vi "校准参数读取.vi"(8 "error in":errorcluster caption="错误输入", 11 "Channel":u16=81 format="%.0x") -> (0 "error out":errorcluster caption="错误输出", 1 "斜率":i32, 2 "截距":i32)   [LabVIEW 2020]
uses:
  D/Program Files (x86)/National Instruments/LabVIEW 2020/user.lib/PCANBasic/PCANBasic.lvlib
panel:
  out "function return 4":u32 format="%.0x"
  out "function return 3":u32 format="%.0x"
  out "function return 2":u32 format="%.0x"
  out "function return":u32 format="%.0x"
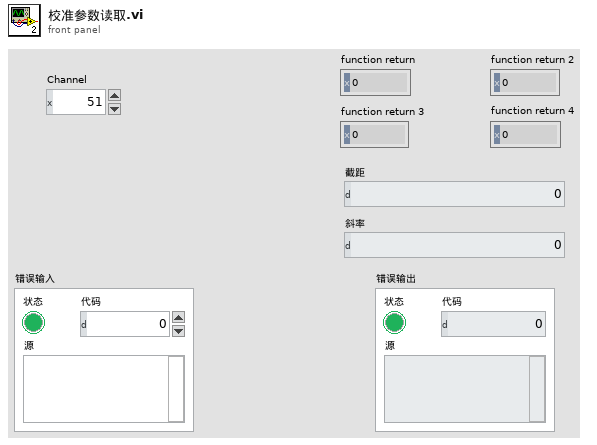
[diagram p1: front panel]
types:
  T1 = cluster{"ID":u32, "MSGTYPE":u8, "DLC":u8, "DATA[0]":u8, "DATA[1]":u8, "DATA[2]":u8, "DATA[3]":u8, "DATA[4]":u8, "DATA[5]":u8, "DATA[6]":u8, "DATA[7]":u8, "DATA[8]":u8, "DATA[9]":u8, "DATA[10]":u8, "DATA[11]":u8, "DATA[12]":u8, "DATA[13]":u8, "DATA[14]":u8, "DATA[15]":u8, "DATA[16]":u8, "DATA[17]":u8, "DATA[18]":u8, "DATA[19]":u8, "DATA[20]":u8, "DATA[21]":u8, "DATA[22]":u8, "DATA[23]":u8, "DATA[24]":u8, "DATA[25]":u8, "DATA[26]":u8, "DATA[27]":u8, "DATA[28]":u8, "DATA[29]":u8, "DATA[30]":u8, "DATA[31]":u8, "DATA[32]":u8, "DATA[33]":u8, "DATA[34]":u8, "DATA[35]":u8, "DATA[36]":u8, "DATA[37]":u8, "DATA[38]":u8, "DATA[39]":u8, "DATA[40]":u8, "DATA[41]":u8, "DATA[42]":u8, "DATA[43]":u8, "DATA[44]":u8, "DATA[45]":u8, "DATA[46]":u8, "DATA[47]":u8, "DATA[48]":u8, "DATA[49]":u8, "DATA[50]":u8, "DATA[51]":u8, "DATA[52]":u8, "DATA[53]":u8, "DATA[54]":u8, "DATA[55]":u8, "DATA[56]":u8, "DATA[57]":u8, "DATA[58]":u8, "DATA[59]":u8, "DATA[60]":u8, "DATA[61]":u8, "DATA[62]":u8, "DATA[63]":u8}
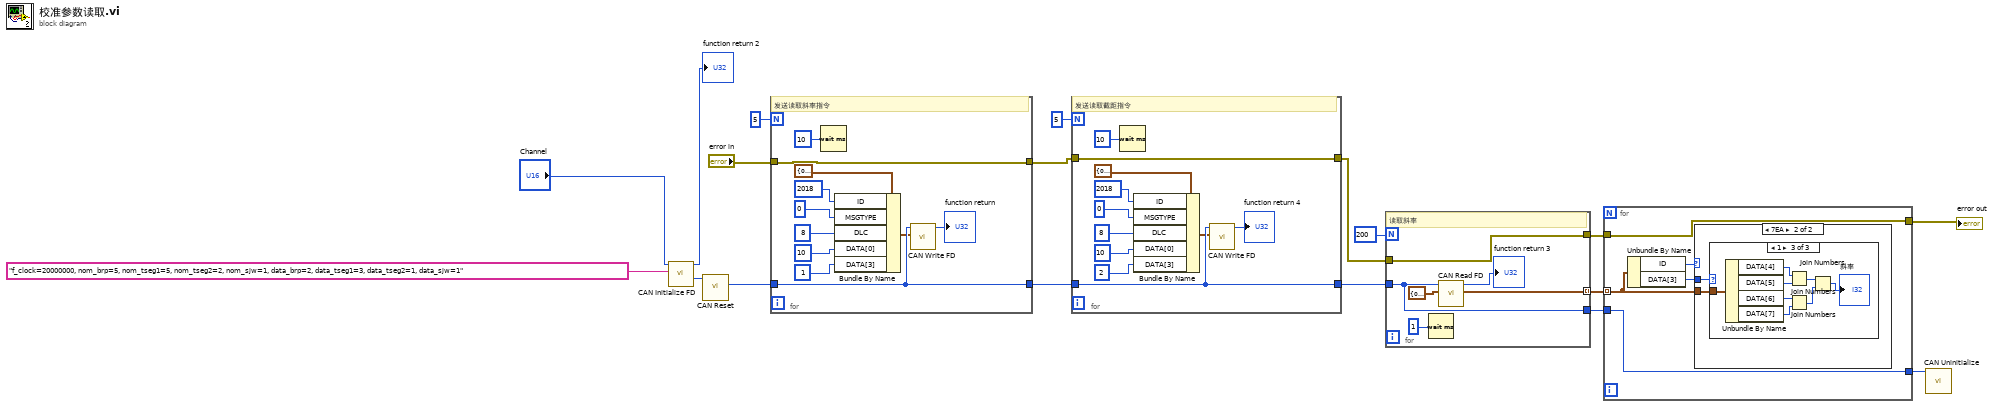
[diagram p0: block diagram]
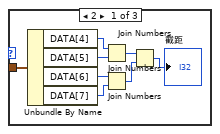
[diagram p3: hidden frame]
diagram:
  n1 = call "CAN Initialize FD.vi"("BitrateFD"="f_clock=20000000, nom_brp=5, nom_tseg1=5, nom_tseg2=2, nom_sjw=1, data_brp=2, data_tseg1=3, data_tseg2=1, data_sjw=1", "Channel"="Channel") -> ("Channel out"=w10:u16, "function return"=→"function return 2":u32)  [unwired: 7 in, 1 out]
  n2 = call "CAN Reset.vi"("Channel in"=w10) -> ("Channel out"=w9:u16)  [unwired: 9 in, 1 out]
  n3 = for {
    N: 5 -> [_]
    tunnel: w9 -> [w26]
    tunnel: [w26] -> w8
    tunnel: "error in" -> [w19]
    tunnel: [w19] -> w4
    # "发送读取斜率指令"
    n4 = Wait (ms)(milliseconds to wait=u32 10 ("等待时间（毫秒）")) -> ()  [unwired: 1 out]
    n5 = Bundle By Name(cluster=T1 {"ID"=0, "MSGTYPE"=0, "DLC"=0, "DATA[0]"=0, "DATA[1]"=0, "DATA[2]"=0, "DATA[3]"=0, "DATA[4]"=0, "DATA[5]"=0, "DATA[6]"=0, "DATA[7]"=0, "DATA[8]"=0, "DATA[9]"=0, "DATA[10]"=0, "DATA[11]"=0, "DATA[12]"=0, "DATA[13]"=0, "DATA[14]"=0, "DATA[15]"=0, "DATA[16]"=0, "DATA[17]"=0, "DATA[18]"=0, "DATA[19]"=0, "DATA[20]"=0, "DATA[21]"=0, "DATA[22]"=0, "DATA[23]"=0, "DATA[24]"=0, "DATA[25]"=0, "DATA[26]"=0, "DATA[27]"=0, "DATA[28]"=0, "DATA[29]"=0, "DATA[30]"=0, "DATA[31]"=0, "DATA[32]"=0, "DATA[33]"=0, "DATA[34]"=0, "DATA[35]"=0, "DATA[36]"=0, "DATA[37]"=0, "DATA[38]"=0, "DATA[39]"=0, "DATA[40]"=0, "DATA[41]"=0, "DATA[42]"=0, "DATA[43]"=0, "DATA[44]"=0, "DATA[45]"=0, "DATA[46]"=0, "DATA[47]"=0, "DATA[48]"=0, "DATA[49]"=0, "DATA[50]"=0, "DATA[51]"=0, "DATA[52]"=0, "DATA[53]"=0, "DATA[54]"=0, "DATA[55]"=0, "DATA[56]"=0, "DATA[57]"=0, "DATA[58]"=0, "DATA[59]"=0, "DATA[60]"=0, "DATA[61]"=0, "DATA[62]"=0, "DATA[63]"=0} ("MessageBuffer"), "ID"=u32 2018, "MSGTYPE"=u8 0, "DLC"=u8 8 ("ID"), "DATA[0]"=u8 10 ("ID"), "DATA[3]"=u8 1) -> (w20:T1)
    n6 = call "CAN Write FD.vi"("MessageBuffer"=w20, "Channel"=w26) -> ("function return"=→"function return":u32)  [unwired: 7 in, 2 out]
  }
  n7 = for {
    N: 5 -> [_]
    tunnel: w8 -> [w37]
    tunnel: [w37] -> w7
    tunnel: w4 -> [w30]
    tunnel: [w30] -> w3
    # "发送读取截距指令"
    n8 = Wait (ms)(milliseconds to wait=u32 10 ("等待时间（毫秒）")) -> ()  [unwired: 1 out]
    n9 = Bundle By Name(cluster=T1 {"ID"=0, "MSGTYPE"=0, "DLC"=0, "DATA[0]"=0, "DATA[1]"=0, "DATA[2]"=0, "DATA[3]"=0, "DATA[4]"=0, "DATA[5]"=0, "DATA[6]"=0, "DATA[7]"=0, "DATA[8]"=0, "DATA[9]"=0, "DATA[10]"=0, "DATA[11]"=0, "DATA[12]"=0, "DATA[13]"=0, "DATA[14]"=0, "DATA[15]"=0, "DATA[16]"=0, "DATA[17]"=0, "DATA[18]"=0, "DATA[19]"=0, "DATA[20]"=0, "DATA[21]"=0, "DATA[22]"=0, "DATA[23]"=0, "DATA[24]"=0, "DATA[25]"=0, "DATA[26]"=0, "DATA[27]"=0, "DATA[28]"=0, "DATA[29]"=0, "DATA[30]"=0, "DATA[31]"=0, "DATA[32]"=0, "DATA[33]"=0, "DATA[34]"=0, "DATA[35]"=0, "DATA[36]"=0, "DATA[37]"=0, "DATA[38]"=0, "DATA[39]"=0, "DATA[40]"=0, "DATA[41]"=0, "DATA[42]"=0, "DATA[43]"=0, "DATA[44]"=0, "DATA[45]"=0, "DATA[46]"=0, "DATA[47]"=0, "DATA[48]"=0, "DATA[49]"=0, "DATA[50]"=0, "DATA[51]"=0, "DATA[52]"=0, "DATA[53]"=0, "DATA[54]"=0, "DATA[55]"=0, "DATA[56]"=0, "DATA[57]"=0, "DATA[58]"=0, "DATA[59]"=0, "DATA[60]"=0, "DATA[61]"=0, "DATA[62]"=0, "DATA[63]"=0} ("MessageBuffer"), "ID"=u32 2018, "MSGTYPE"=u8 0, "DLC"=u8 8 ("ID"), "DATA[0]"=u8 10 ("ID"), "DATA[3]"=u8 2) -> (w31:T1)
    n10 = call "CAN Write FD.vi"("MessageBuffer"=w31, "Channel"=w37) -> ("function return"=→"function return 4":u32)  [unwired: 7 in, 2 out]
  }
  n11 = for {
    N: 200 -> [_]
    tunnel: w7 -> [w45]
    tunnel: [w44] -> w16 mode=indexing
    tunnel: [w45] -> w15
    tunnel: w3 -> [w41]
    tunnel: [w41] -> w2
    # "读取斜率"
    n12 = Wait (ms)(milliseconds to wait=u32 1 ("等待时间（毫秒）")) -> ()  [unwired: 1 out]
    n13 = call "CAN Read FD.vi"("MessageBuffer"=T1 {"ID"=0, "MSGTYPE"=0, "DLC"=0, "DATA[0]"=0, "DATA[1]"=0, "DATA[2]"=0, "DATA[3]"=0, "DATA[4]"=0, "DATA[5]"=0, "DATA[6]"=0, "DATA[7]"=0, "DATA[8]"=0, "DATA[9]"=0, "DATA[10]"=0, "DATA[11]"=0, "DATA[12]"=0, "DATA[13]"=0, "DATA[14]"=0, "DATA[15]"=0, "DATA[16]"=0, "DATA[17]"=0, "DATA[18]"=0, "DATA[19]"=0, "DATA[20]"=0, "DATA[21]"=0, "DATA[22]"=0, "DATA[23]"=0, "DATA[24]"=0, "DATA[25]"=0, "DATA[26]"=0, "DATA[27]"=0, "DATA[28]"=0, "DATA[29]"=0, "DATA[30]"=0, "DATA[31]"=0, "DATA[32]"=0, "DATA[33]"=0, "DATA[34]"=0, "DATA[35]"=0, "DATA[36]"=0, "DATA[37]"=0, "DATA[38]"=0, "DATA[39]"=0, "DATA[40]"=0, "DATA[41]"=0, "DATA[42]"=0, "DATA[43]"=0, "DATA[44]"=0, "DATA[45]"=0, "DATA[46]"=0, "DATA[47]"=0, "DATA[48]"=0, "DATA[49]"=0, "DATA[50]"=0, "DATA[51]"=0, "DATA[52]"=0, "DATA[53]"=0, "DATA[54]"=0, "DATA[55]"=0, "DATA[56]"=0, "DATA[57]"=0, "DATA[58]"=0, "DATA[59]"=0, "DATA[60]"=0, "DATA[61]"=0, "DATA[62]"=0, "DATA[63]"=0}, "Channel"=w45) -> ("MessageBuffer out"=w44:T1, "function return"=→"function return 3":u32)  [unwired: 6 in, 2 out]
  }
  n14 = for {
    tunnel: w16 -> [w50] mode=indexing
    tunnel: [w51] -> w14
    tunnel: w15 -> [w51]
    tunnel: w2 -> [w47]
    tunnel: [w47] -> w1
    n15 = Unbundle By Name(w50) -> ("ID"=w49:u32, "DATA[3]"=w48:u8)
    n16 = case shown="7EA" w49 {
      tunnel: w50 -> [_ w53]
      tunnel: w48 -> [_ w52]
      frame 0, Default {
      }
      frame 2026 {
        n17 = case shown="1" w52 {
          tunnel: w53 -> [w54 _ w69]
          frame 2 {
            n18 = Unbundle By Name(w54) -> ("DATA[4]"=w61:u8, "DATA[5]"=w60:u8, "DATA[6]"=w59:u8, "DATA[7]"=w58:u8)
            n19 = Join Numbers(hi=w61, lo=w60) -> ((hi.lo)=w56:u16)
            n20 = Join Numbers(hi=w59, lo=w58) -> ((hi.lo)=w57:u16)
            n21 = Join Numbers(hi=w56, lo=w57) -> ((hi.lo)=→"截距":u32)
          }
          frame 3, Default {
          }
          frame 1 {
            n22 = Unbundle By Name(w69) -> ("DATA[4]"=w68:u8, "DATA[5]"=w67:u8, "DATA[6]"=w66:u8, "DATA[7]"=w65:u8)
            n23 = Join Numbers(hi=w68, lo=w67) -> ((hi.lo)=w63:u16)
            n24 = Join Numbers(hi=w66, lo=w65) -> ((hi.lo)=w64:u16)
            n25 = Join Numbers(hi=w63, lo=w64) -> ((hi.lo)=→"斜率":u32)
          }
        }
      }
    }
  }
  "error out" <- w1
  n26 = call "CAN Uninitialize.vi"("Channel"=w14) -> ()  [unwired: 10 in, 1 out]
